vi "xy_weight_height_2.vi"() -> ()   [LabVIEW 2021]
uses:
  <vilib>/Utility/file.llb/Read Delimited Spreadsheet (string).vi
  <vilib>/Analysis/NI_AALBase.lvlib
panel:
  out "Weight Distribution":T1(graph)
  out "Height Distribution":T2(graph)
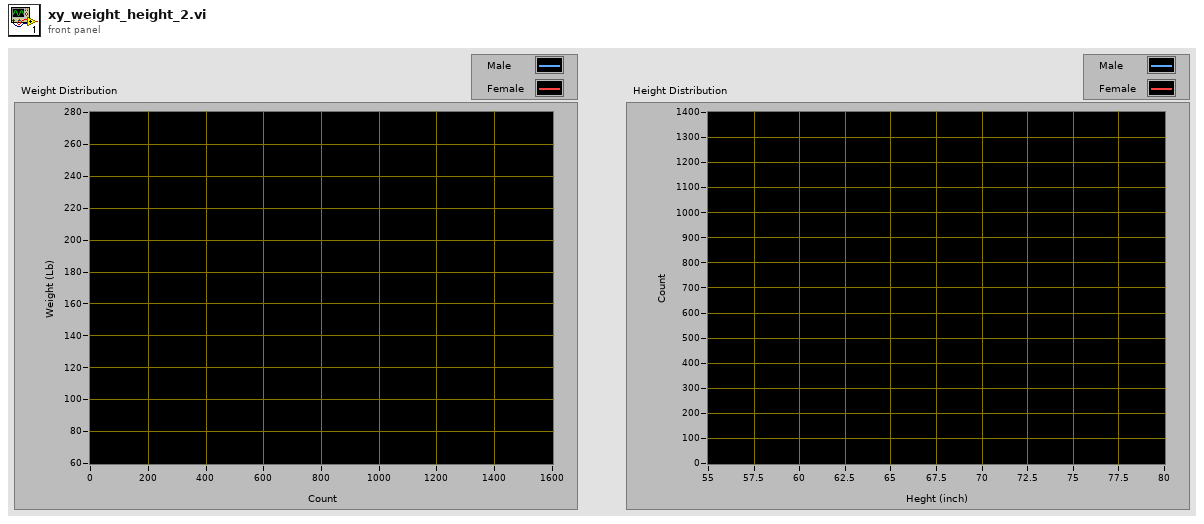
[diagram p1: front panel]
types:
  T1 = cluster{"Histogram: h(x)":i32[], "X Values":dbl[]}[]
  T2 = cluster{"X Values":dbl[], "Histogram: h(x)":i32[]}[]
  T3 = cluster{"X Values":dbl[], "Histogram: h(x)":i32[]}
  T4 = cluster{"Histogram: h(x)":i32[], "X Values":dbl[]}
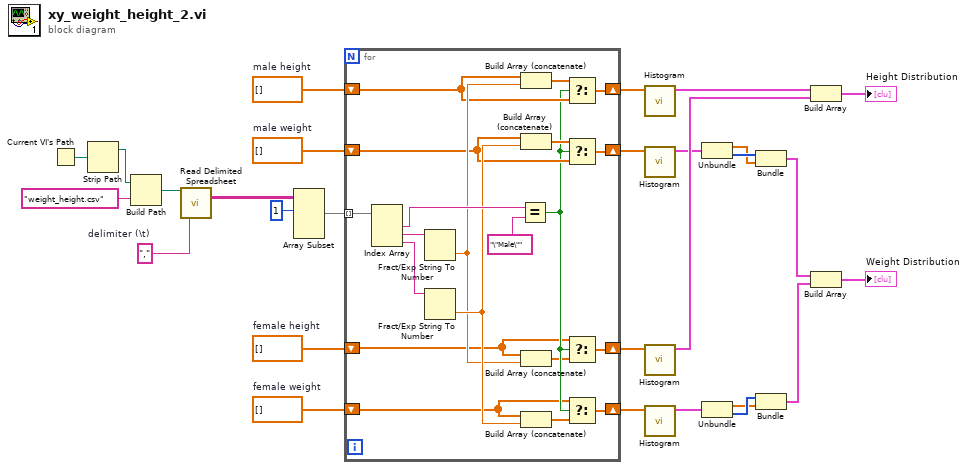
[diagram p0: block diagram]
diagram:
  w17 = dbl[] []  # female weight
  w18 = dbl[] []  # female height
  w19 = dbl[] []  # male weight
  w20 = dbl[] []  # male height
  w24 = ","  # delimiter (\t)
  n1 = Current VI's Path() -> (path=w28:path)
  n2 = Strip Path(path=w28) -> (stripped path=w27:path)  [unwired: 1 out]
  n3 = Build Path(base path=w27, name or relative path="weight_height.csv") -> (appended path=w25:path)
  n4 = call-poly <vilib>:"Read Delimited Spreadsheet.vi"("file path (dialog if empty)"=w25, "delimiter (\\t)"=w24) -> ("all rows"=w23:string[][])  [unwired: 8 in, 5 out]
  n5 = Array Subset(array=w23, index (row)=1 ("index")) -> (w21:string[][])  [unwired: 3 in]
  n6 = for {
    tunnel: w21 -> [w48] mode=indexing
    shift-right: [w43] -> w16
    shift-left: w20 -> [w37]
    shift-right: [w40] -> w15
    shift-left: w19 -> [w36]
    shift-right: [w29] -> w14
    shift-left: w18 -> [w34]
    shift-right: [w30] -> w13
    shift-left: w17 -> [w33]
    n7 = Index Array(array=w48) -> (element #1=w47:string, element #2=w45:string, element #3=w41:string)  [unwired: 3 in]
    n8 = Fract/Exp String To Number(string=w45) -> (number=w38:dbl)  [unwired: 3 in, 1 out]
    n9 = Fract/Exp String To Number(string=w41) -> (number=w39:dbl)  [unwired: 3 in, 1 out]
    n10 = Equal?(x=w47, y="\"Male\"") -> (x = y?=w35:bool)
    n11 = Build Array (concatenate)(w37, w38) -> (w44:dbl[])
    n12 = Build Array (concatenate)(w36, w39) -> (w42:dbl[])
    n13 = Build Array (concatenate)(w34, w38) -> (w32:dbl[])
    n14 = Build Array (concatenate)(w33, w39) -> (w31:dbl[])
    n15 = Select(t=w44, s=w35, f=w37) -> (s? t:f=w43:dbl[])
    n16 = Select(t=w42, s=w35, f=w36) -> (s? t:f=w40:dbl[])
    n17 = Select(t=w34, s=w35, f=w32) -> (s? t:f=w29:dbl[])
    n18 = Select(t=w33, s=w35, f=w31) -> (s? t:f=w30:dbl[])
  }
  n19 = call <vilib>:"Histogram.vi"("X"=w16) -> ("Histogram Graph"=w12:T3)  [unwired: 7 in, 3 out]
  n20 = call <vilib>:"Histogram.vi"("X"=w15) -> ("Histogram Graph"=w9:T3)  [unwired: 7 in, 3 out]
  n21 = call <vilib>:"Histogram.vi"("X"=w14) -> ("Histogram Graph"=w11:T3)  [unwired: 7 in, 3 out]
  n22 = call <vilib>:"Histogram.vi"("X"=w13) -> ("Histogram Graph"=w5:T3)  [unwired: 7 in, 3 out]
  n23 = Unbundle(w9) -> ("X Values"=w7:dbl[], "Histogram: h(x)"=w8:i32[])
  n24 = Unbundle(w5) -> ("X Values"=w3:dbl[], "Histogram: h(x)"=w4:i32[])
  n25 = Bundle("Histogram: h(x)"=w8, "X Values"=w7) -> (w6:T4)  [unwired: 1 in]
  n26 = Bundle("Histogram: h(x)"=w4, "X Values"=w3) -> (w2:T4)  [unwired: 1 in]
  n27 = Build Array(w12, w11) -> (→"Height Distribution":T2)
  n28 = Build Array(w6, w2) -> (→"Weight Distribution":T1)
